vi "EQC load ChipIDs.vi"(8 "EQ Leak3 folder path":path caption="Leakage 3 EQ", 9 "EQ Leak2 folder path":path caption="Leakage 2 EQ", 10 "EQ Leak1 folder path":path caption="Leakage 1 EQ", 11 "EQ Leak0 folder path":path caption="Leakage 0 EQ") -> (2 "ChipID list 1i2":string[](array[string]))   [LabVIEW 2015, in "VIPM2.lvlib"]
doc: "Load ChipID list from main EQ summary file."
uses:
  VIPM2.lvlib
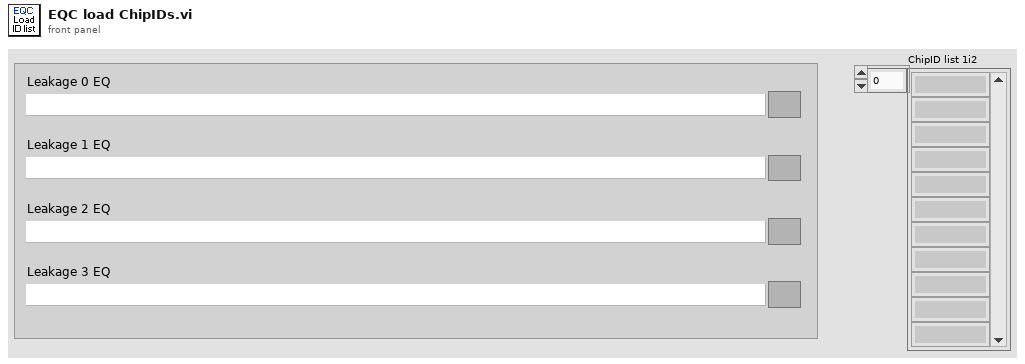
[diagram p1: front panel]
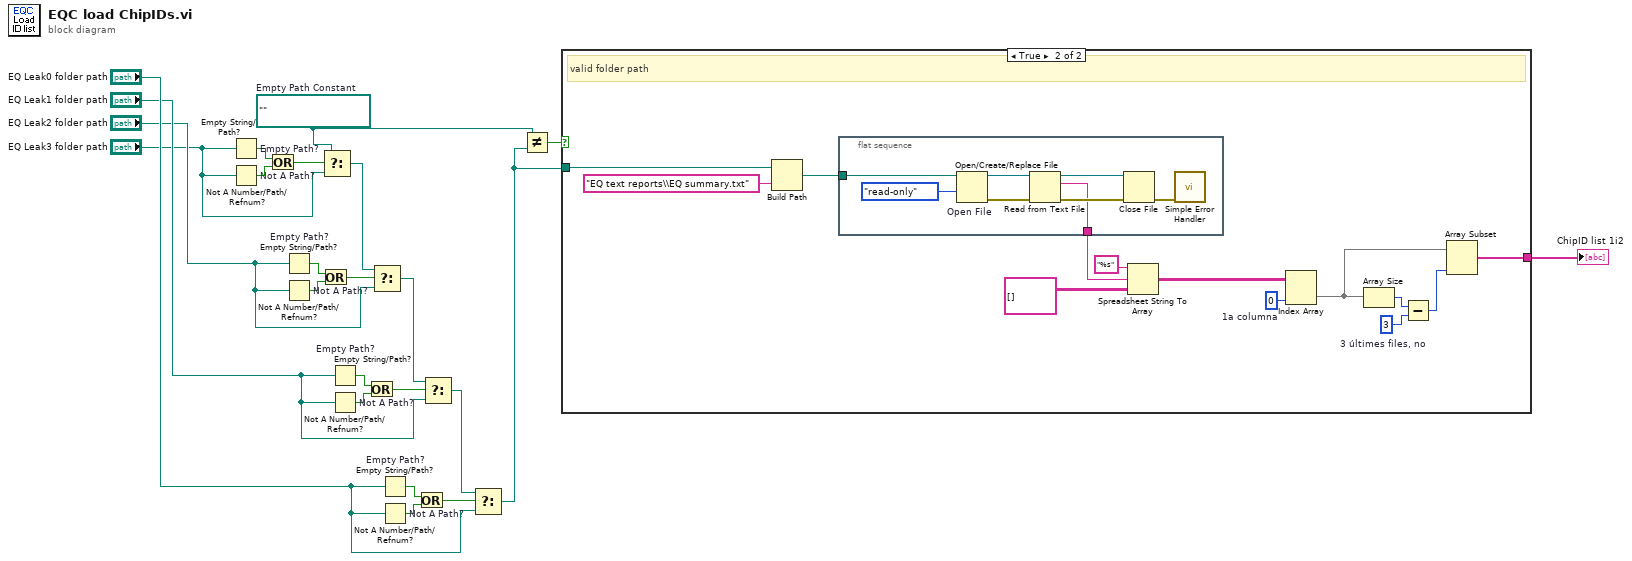
[diagram p0: block diagram]
diagram:
  w4 = path ""  # Empty Path Constant
  n1 = Empty String/Path? "Empty Path?"(string/path="EQ Leak3 folder path") -> (empty?=w13:bool)
  n2 = Not A Number/Path/Refnum? "Not A Path?"(number/path/refnum="EQ Leak3 folder path") -> (NaN/Path/Refnum?=w12:bool)
  n3 = Or(x=w13, y=w12) -> (x .or. y?=w14:bool)
  n4 = Empty String/Path? "Empty Path?"(string/path="EQ Leak2 folder path") -> (empty?=w16:bool)
  n5 = Not A Number/Path/Refnum? "Not A Path?"(number/path/refnum="EQ Leak2 folder path") -> (NaN/Path/Refnum?=w17:bool)
  n6 = Or(x=w16, y=w17) -> (x .or. y?=w15:bool)
  n7 = Select(t=w4, s=w14, f="EQ Leak3 folder path") -> (s? t:f=w5:path)
  n8 = Empty String/Path? "Empty Path?"(string/path="EQ Leak1 folder path") -> (empty?=w19:bool)
  n9 = Not A Number/Path/Refnum? "Not A Path?"(number/path/refnum="EQ Leak1 folder path") -> (NaN/Path/Refnum?=w18:bool)
  n10 = Or(x=w19, y=w18) -> (x .or. y?=w20:bool)
  n11 = Select(t=w5, s=w15, f="EQ Leak2 folder path") -> (s? t:f=w8:path)
  n12 = Empty String/Path? "Empty Path?"(string/path="EQ Leak0 folder path") -> (empty?=w22:bool)
  n13 = Not A Number/Path/Refnum? "Not A Path?"(number/path/refnum="EQ Leak0 folder path") -> (NaN/Path/Refnum?=w23:bool)
  n14 = Or(x=w22, y=w23) -> (x .or. y?=w21:bool)
  n15 = Select(t=w8, s=w20, f="EQ Leak1 folder path") -> (s? t:f=w10:path)
  n16 = Select(t=w10, s=w21, f="EQ Leak0 folder path") -> (s? t:f=w2:path)
  n17 = Not Equal?(x=w4, y=w2) -> (x != y?=w3:bool)
  n18 = case shown="True" w3 {
    tunnel: w2 -> [_ w35]
    tunnel: [_ w24] -> w1
    frame False {
      # "no folder path"
    }
    frame True {
      w25 = 0  # 1a columna
      w30 = 3  # 3 últimes files, no
      # "valid folder path"
      n19 = Build Path(base path=w35, name or relative path="EQ text reports\\EQ summary.txt") -> (appended path=w31:path)
      n20 = flat-sequence {
        tunnel: [w39] -> w32
        tunnel: w31 -> [w37]
        frame #0 {
          n21 = Open/Create/Replace File "Open File"(file path (use dialog)=w37, access (0:read/write)=enum16{"read/write", "read-only", "write-only"}."read-only") -> (refnum out=w43:refnum<file>, error out=w42:errorcluster)  [unwired: 4 in, 1 out]
          n22 = Read from Text File(file (use dialog)=w43, error in=w42) -> (refnum out=w41:refnum<file>, text=w39:string, error out=w40:errorcluster)  [unwired: 2 in, 1 out]
          n23 = Close File(refnum=w41, error in=w40) -> (error out=w38:errorcluster)  [unwired: 1 out]
          n24 = call <vilib>:"Simple Error Handler.vi"("error in (no error)"=w38) -> ()  [unwired: 4 in, 5 out]
        }
      }
      n25 = Spreadsheet String To Array(format string="%s", spreadsheet string=w32, array type (2D Dbl)=string[][] []) -> (array=w28:string[][])  [unwired: 1 in]
      n26 = Index Array "Index Array"(array=w28, index (col)=w25) -> (element=w27:string[])  [unwired: 1 in]
      n27 = Array Size(array=w27) -> (size(s)=w26:i32)
      n28 = Subtract(x=w26, y=w30) -> (x-y=w29:i32)
      n29 = Array Subset "Array Subset"(array=w27, length=w29) -> (w24:string[])  [unwired: 1 in]
    }
  }
  "ChipID list 1i2" <- w1
